vi "Single Z Ramp Approach Descriptor.vi"() -> ()   [LabVIEW 2013]
panel:
  out "Experimental VI Reference":refnum<vi>
  out "Experimental VI Description":string
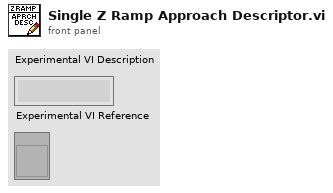
[diagram p1: front panel]
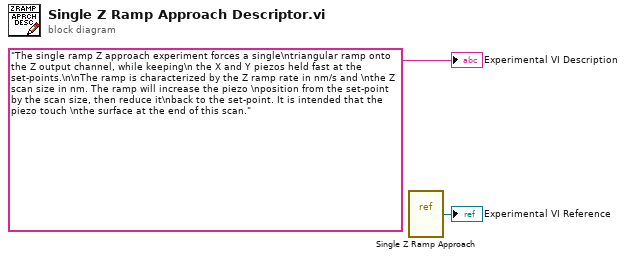
[diagram p0: block diagram]
diagram:
  n1 = vi-ref "Single Z Ramp Approach.vi"() -> (→"Experimental VI Reference":refnum<vi>)
  "Experimental VI Description" <- "The single ramp Z approach experiment forces a single\ntriangular ramp onto the Z output channel, while keeping\n the X and Y piezos held fast at the set-points.\n\nThe ramp is characterized by the Z ramp rate in nm/s and \nthe Z scan size in nm. The ramp will increase the piezo \nposition from the set-point by the scan size, then reduce it\nback to the set-point. It is intended that the piezo touch \nthe surface at the end of this scan."
